vi "[GV]_GPS Raw_Lat.vi"() -> ()   [LabVIEW 2016]
panel:
  out "GPS Raw_Lat":dbl format="%.8f"
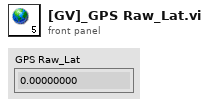
[diagram p1: front panel]
diagram:
